vi "Host_17.vi"() -> ()   [LabVIEW 2017]
panel:
  out "Feedback Load Torque":dbl
  out "Feedback Duty Cycle":dbl
  in  "?":bool
  in  "Load Torque":dbl(slide) scale=-0.2..0.2
  in  "Duty Cycle":dbl(slide) scale=0.0..100.0
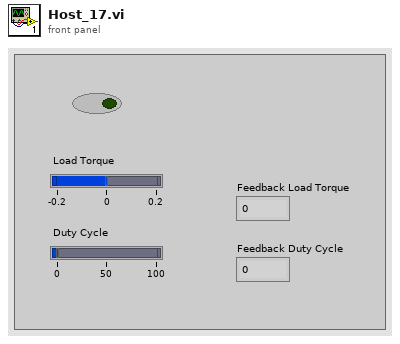
[diagram p1: front panel]
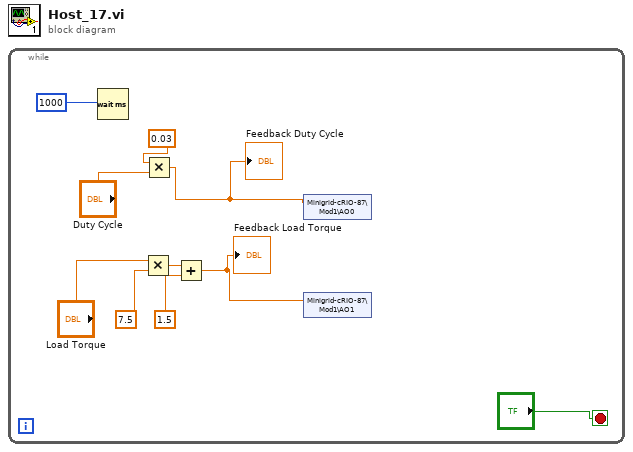
[diagram p0: block diagram]
diagram:
  n1 = while {
    stop <- "?" stop-if-true
    n2 = Wait (ms)(milliseconds to wait=1000) -> ()  [unwired: 1 out]
    n3 = Multiply(x="Load Torque", y=7.5) -> (x*y=w5:dbl)
    n4 = Multiply(x=0.03, y="Duty Cycle") -> (x*y=w6:dbl)
    "Feedback Duty Cycle" <- w6
    n5 = Add(x=w5, y=1.5) -> (x+y=w1:dbl)
    "Feedback Load Torque" <- w1
    n6 = shared-variable "Minigrid-cRIO-87\\Mod1\\AO0"(w6) -> ()  [unwired: 1 in, 1 out]
    n7 = shared-variable "Minigrid-cRIO-87\\Mod1\\AO1"(w1) -> ()  [unwired: 1 in, 1 out]
  }
